vi "Test Name of Test Case in Result when Creating Suite from Test Case.vi"(8 "error in (no error)":errorcluster, 11 "Test Case In":refnum<class "LUnit Test Suite Tests.lvclass">) -> (0 "error out":errorcluster, 3 "Test Case Out":refnum<class "LUnit Test Suite Tests.lvclass">)   [LabVIEW 2020, in "LUnit Test Suite Tests.lvclass"]
uses:
  LUnit Test Suite Tests.lvclass
  C:/Program Files (x86)/National Instruments/LabVIEW 2020/vi.lib/Astemes/LUnit/Test Case.lvclass
  LUnit Test Case Tests/LUnit Test Case V2 Test Double/LUnit Test Case V2 Test Double.lvclass
  C:/Git/astemes-lunit/source/Rewrite Project/LUnit Test Case/LUnit Test Case V2.lvclass
  <vilib>/Astemes/LUnit/Test Case.lvclass/Test Case.ctl
  b74e4934-f044-4222-b3dd-fc90e6c1bd4f.vi
  <vilib>/Astemes/LUnit/Palette/Pass.vi
  <vilib>/Astemes/LUnit/Palette/Fail.vi
  <vilib>/Astemes/LUnit/Compare Variants.vi
  <vilib>/Astemes/LUnit/Describe Comparison.vi
  <vilib>/Astemes/LUnit/Set Assertion Type.vi
  <vilib>/Astemes/LUnit/Add test result.vi
  <vilib>/Astemes/LUnit/Variant to string.vi
  <vilib>/Astemes/LUnit/LUnit Record Assertion Result.vi
  <vilib>/Astemes/LUnit/LUnit Aggregate Assertion Results.vi
  <vilib>/Astemes/LUnit/Method Result/LUnit Merge Status.vi
  <vilib>/Astemes/LUnit/LUnit Concatenate result strings.vi
  <vilib>/Utility/Data Type/Get Type Information.vi
  LUnit Test Suite/LUnit Test Suite V2.lvclass
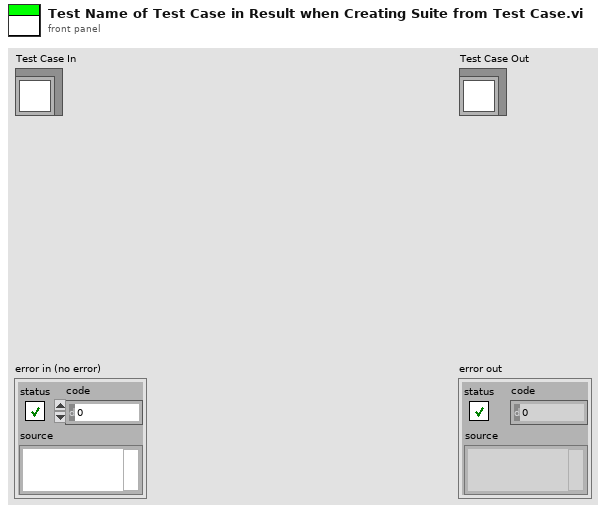
[diagram p1: front panel]
types:
  T1 = typedef "Result.lvlib/Result.ctl" = cluster{"Name":string, "Message":string, "Description":string, "Status":T2, "Result Type":T3, "Execution Time":dbl}
  T2 = typedef "Result.lvlib/Status.ctl" = enum16{"", "Passed", "Failed", "Error", "Skipped", "Setup Error", "Broken", "Teardown Error"}
  T3 = typedef "Result.lvlib/Type.ctl" = enum16{"Method", "Case", "Suite", "Pass", "Fail", "Skip", "Pass if", "Fail if", "Pass if Error", "Fail if Error", "Pass if Equal", "Fail if Equal"}
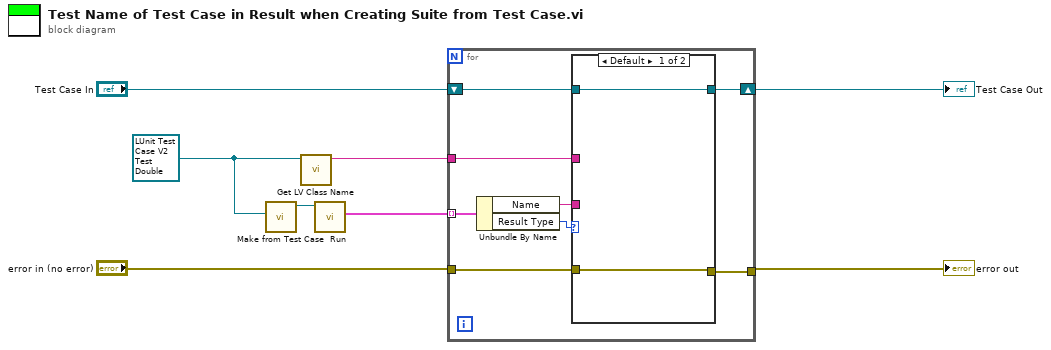
[diagram p0: block diagram]
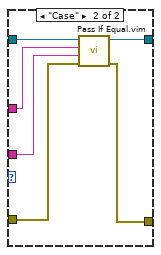
[diagram p2: hidden frame]
diagram:
  w7 = refnum<class "LUnit Test Case V2 Test Double.lvclass"> refnum ("LUnit Test Case V2 Test Double.lvclass")
  n1 = call "Make from Test Case.vi"("LUnit Test Case"=w7) -> ("LUnit Test Suite V2 out"=w8:refnum<class "LUnit Test Suite V2.lvclass">)  [unwired: 9 in, 1 out]
  n2 = call <vilib>:"Get LV Class Name.vi"("object"=w7) -> ("class name"=w1:string)  [unwired: 9 in, 1 out]
  n3 = call-dynamic "Run.vi"("Run in"=w8) -> ("Results"=w6:T1[])  [unwired: 9 in, 1 out]
  n4 = for {
    tunnel: w6 -> [w16] mode=indexing
    tunnel: "error in (no error)" -> [w15]
    tunnel: [w13] -> w3
    shift-right: [w12] -> w2
    shift-left: "Test Case In" -> [w14]
    tunnel: w1 -> [w11]
    n5 = Unbundle By Name(w16) -> ("Name"=w10:string, "Result Type"=w9:T3)
    n6 = case shown="Default" w9 {
      tunnel: w15 -> [w17 w24]
      tunnel: w14 -> [w18 w23]
      tunnel: [w17 w22] -> w13
      tunnel: [w18 w21] -> w12
      tunnel: w11 -> [_ w20]
      tunnel: w10 -> [_ w19]
      frame Default {
      }
      frame "Case" {
        n7 = call "Pass If Equal.vim"("error in (no error)"=w24, "Actual"=w19, "Expected"=w20, "LUnit Test Case In"=w23) -> ("error out"=w22:errorcluster, "LUnit Test Case Out"=w21:refnum<class "LUnit Test Suite Tests.lvclass">)  [unwired: 6 in]
      }
    }
  }
  "error out" <- w3
  "Test Case Out" <- w2
